vi "getImageQualityforCompression.vi"(11 "compression rate":dbl) -> (3 "quality":i16)   [LabVIEW 2011]
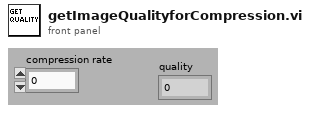
[diagram p1: front panel]
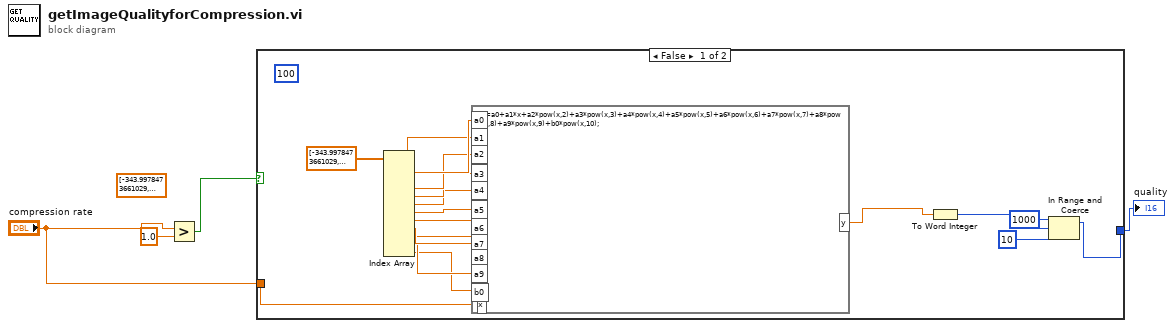
[diagram p0: block diagram]
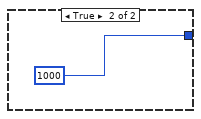
[diagram p2: hidden frame]
diagram:
  (unwired) dbl[] [-343.9978473661029, 17813.381169421064, -100835.71805513835, 44542.45550528182, 2234584.9420572105, -12046109.081565328, 31302820.72776386, -47078728.7976436, 41729570.09482816, -20266318.49339796, 4164004.504123382] ("Array 3")
  n1 = Greater?(x="compression rate", y=1.0) -> (0:w2:bool)
  n2 = case shown="False" w2 {
    tunnel: "compression rate" -> [w6 _]
    tunnel: [w5 i16 1000 ("upper limit")] -> w1
    frame False {
      (unwired) 100
      n3 = Index Array(array=dbl[] [-343.9978473661029, 17813.381169421064, -100835.71805513835, 44542.45550528182, 2234584.9420572105, -12046109.081565328, 31302820.72776386, -47078728.7976436, 41729570.09482816, -20266318.49339796, 4164004.504123382] ("Array 3")) -> (element #1=w22:dbl, element #2=w21:dbl, element #3=w20:dbl, element #4=w19:dbl, element #5=w18:dbl, element #6=w17:dbl, element #7=w16:dbl, element #8=w15:dbl, element #9=w14:dbl, element #10=w13:dbl, element #11=w12:dbl)  [unwired: 11 in]
      n4 = formula code="y=a0+a1*x+a2*pow(x,2)+a3*pow(x,3)+a4*pow(x,4)+a5*pow(x,5)+a6*pow(x,6)+a7*pow(x,7)+a8*pow(x,8)+a9*pow(x,9)+b0*pow(x,10);"("a0"=w22, "a1"=w21, "a2"=w20, "a3"=w19, "a4"=w18, "a5"=w17, "x"=w6, "a6"=w16, "a7"=w15, "a8"=w14, "a9"=w13, "b0"=w12) -> ("y"=w10:dbl)
      n5 = To Word Integer(number=w10) -> (16bit integer=w7:i16)
      n6 = In Range and Coerce(upper limit=i16 1000, x=w7, lower limit=i16 10) -> (coerced(x)=w5:i16)  [unwired: 1 out]
    }
    frame True {
    }
  }
  "quality" <- w1
